vi "GetFileDatafromIndex.vi"(8 "Error In":errorcluster, 10 "Temperature File":dbl[][](array[numeric]) format="%0.3f", 11 "DuplicateFilteredIndex":u32) -> (0 "Error Out":errorcluster, 1 "FreezeAbsTime":timestamp, 2 "FreezeFileName":string, 3 "FreezeTemperature":dbl format="%#_13g", 5 "Peak index":u32)   [LabVIEW 2013]
uses:
  DB/ConfDB.ctl
  DB/ConfEnum.ctl
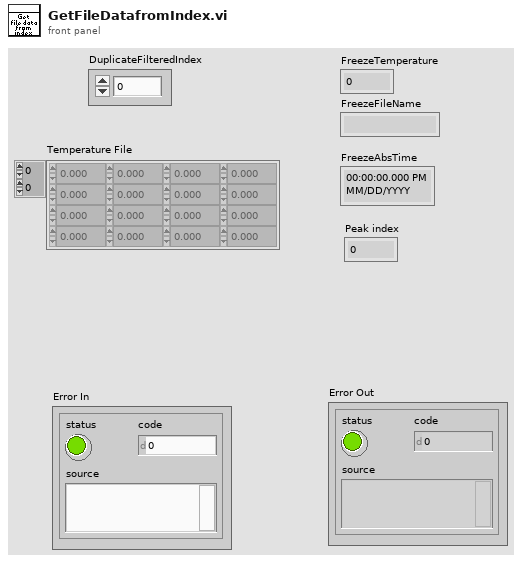
[diagram p1: front panel]
types:
  T1 = typedef "ConfEnum.ctl" = enum16{"Init", "GetConfDB", "WriteConfDB", "Configure DB"}
  T2 = typedef "ConfDB.ctl" = cluster{"NumberOfImages":i32, "NoImages2SaveAroundFreeze":i32, "Path":path, "NameOfPartialFile":string, "StartIndex":i32, "NumberOfStdTol":i32, "Detla t (sec)":i32, "Number of images for baseline":i32, "Temperature File Name":string, "Score":dbl, "Index number of Files":i32[], "End Index":i32}
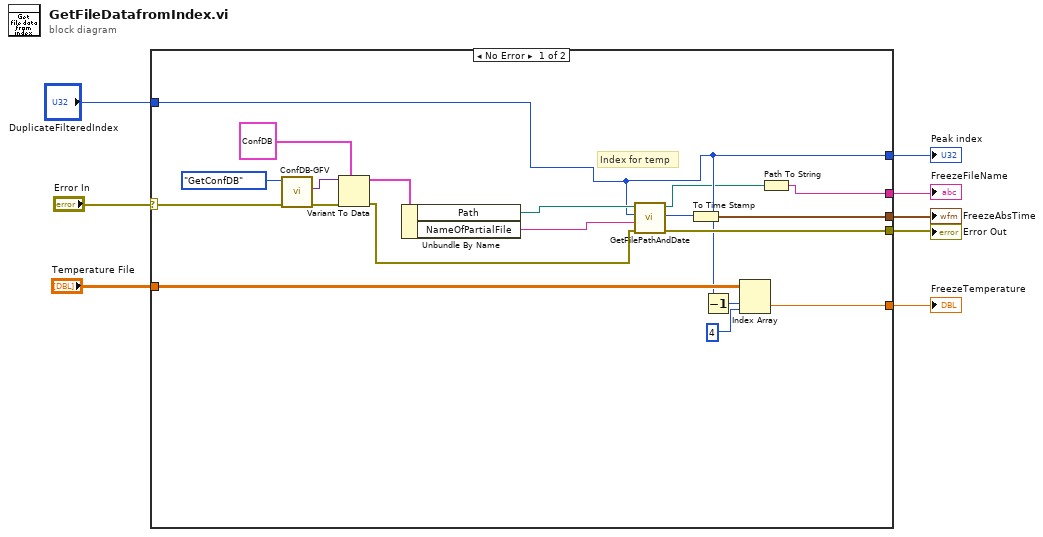
[diagram p0: block diagram]
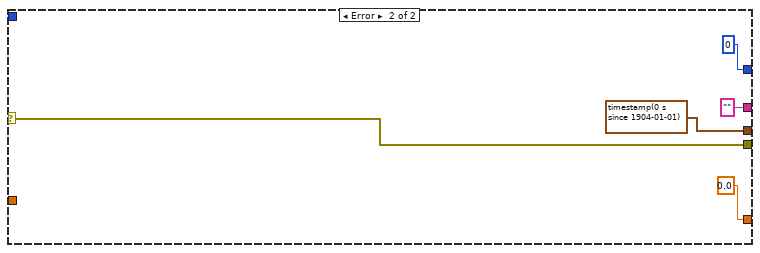
[diagram p2: hidden frame]
diagram:
  n1 = case shown="No Error" "Error In" {
    selector: "Error In" -> [w21 w32]
    tunnel: "DuplicateFilteredIndex" -> [w11 _]
    tunnel: [w17 w32] -> w6
    tunnel: [w18 timestamp(0 s since 1904-01-01)] -> w5
    tunnel: [w9 "" ("name")] -> w4
    tunnel: [w11 0] -> w3
    tunnel: [w13 0.0] -> w2
    tunnel: "Temperature File" -> [w12 _]
    frame No Error {
      # "Index for temp"
      n2 = call "ConfDB-GFV.vi"("error in (no error)"=w21, "Command In"=ConfEnum."GetConfDB") -> ("error out"=w24:errorcluster, "Data out"=w25:variant)  [unwired: 8 in]
      n3 = Variant To Data(error in=w24, type=T2 {"NumberOfImages"=0, "NoImages2SaveAroundFreeze"=0, "Path"=path "", "NameOfPartialFile"="", "StartIndex"=0, "NumberOfStdTol"=0, "Detla t (sec)"=0, "Number of images for baseline"=0, "Temperature File Name"="", "Score"=0.0, "Index number of Files"=[], "End Index"=0} ("ConfDB"), Variant=w25) -> (data=w26:T2, error out=w20:errorcluster)
      n4 = Unbundle By Name(w26) -> ("Path"=w16:path, "NameOfPartialFile"=w27:string)
      n5 = call "GetFilePathAndDate.vi"("error in (no error)"=w20, "String"=w27, "Index"=w11, "Path"=w16) -> ("error out"=w17:errorcluster, "creation date"=w19:u32, "file out"=w10:path)  [unwired: 5 in]
      n6 = To Time Stamp(1:w19) -> (0:w18:timestamp)
      n7 = Decrement(x=w11) -> (x-1=w15:u32)
      n8 = Index Array(array=w12, index (row)=w15, index (col)=4 ("disabled index (col)")) -> (element=w13:dbl)
      n9 = Path To String(path=w10) -> (string=w9:string)
    }
    frame Error {
    }
  }
  "Error Out" <- w6
  "FreezeTemperature" <- w2
  "FreezeFileName" <- w4
  "FreezeAbsTime" <- w5
  "Peak index" <- w3
